vi "MH_WriteTestPTUFile.vi"(8 "entrée d'erreur":errorcluster) -> (0 "sortie d'erreur":errorcluster, 3 "refnum Out":refnum<file>)   [LabVIEW 2019]
panel:
  out "Tableau":u32[](array[numeric])
  in  "Path":path
  in  "TagArray":T1(array[cluster])=[{"TagIdent"="File_GUID", "TagIndex"=-1, "TagType"=1073872895, "TagValue"=40, "TagAuxData"="{197B8EE0-02FE-45EA-A6B5-3F8BBDE2D882}\u0000\u0000"}, {"TagIdent"="File_AssuredContent", "TagIndex"=-1, "TagType"=1073872895, "TagValue"=32, "TagAuxData"="MultiHarp: HWSETG SWSETG\u0000\u0000\u0000\u0000\u0000\u0000\u0000\u0000"}, {"TagIdent"="CreatorSW_ContentVersion", "TagIndex"=-1, "TagType"=1073872895, "TagValue"=8, "TagAuxData"="1.0\u0000\u0000\u0000\u0000\u0000"}, {"TagIdent"="CreatorSW_Name", "TagIndex"=-1, "TagType"=1073872895, "TagValue"=16, "TagAuxData"="MultiHarp AcqUI\u0000"}, {"TagIdent"="CreatorSW_Version", "TagIndex"=-1, "TagType"=1073872895, "TagValue"=8, "TagAuxData"="3.0.0.0\u0000"}, {"TagIdent"="File_CreatingTime", "TagIndex"=-1, "TagType"=553648136, "TagValue"=4676398420989345414, "TagAuxData"=""}, {"TagIdent"="File_Comment", "TagIndex"=-1, "TagType"=1073872895, "TagValue"=8, "TagAuxData"="T2 Mode\u0000"}, {"TagIdent"="Measurement_Mode", "TagIndex"=-1, "TagType"=268435464, "TagValue"=2, "TagAuxData"=""}, {"TagIdent"="Measurement_SubMode", "TagIndex"=-1, "TagType"=268435464, "TagValue"=0, "TagAuxData"=""}, {"TagIdent"="TTResult_StopReason", "TagIndex"=-1, "TagType"=268435464, "TagValue"=0, "TagAuxData"=""}, {"TagIdent"="Fast_Load_End", "TagIndex"=-1, "TagType"=-65528, "TagValue"=0, "TagAuxData"=""}, {"TagIdent"="TTResultFormat_TTTRRecType", "TagIndex"=-1, "TagType"=268435464, "TagValue"=66055, "TagAuxData"=""}, {"TagIdent"="TTResultFormat_BitsPerRecord", "TagIndex"=-1, "TagType"=268435464, "TagValue"=32, "TagAuxData"=""}, {"TagIdent"="MeasDesc_BinningFactor", "TagIndex"=-1, "TagType"=268435464, "TagValue"=32, "TagAuxData"=""}, {"TagIdent"="MeasDesc_Offset", "TagIndex"=-1, "TagType"=268435464, "TagValue"=0, "TagAuxData"=""}, {"TagIdent"="MeasDesc_AcquisitionTime", "TagIndex"=-1, "TagType"=268435464, "TagValue"=900000, "TagAuxData"=""}, {"TagIdent"="MeasDesc_StopAt", "TagIndex"=-1, "TagType"=268435464, "TagValue"=4294967295, "TagAuxData"=""}, {"TagIdent"="MeasDesc_StopOnOvfl", "TagIndex"=-1, "TagType"=8, "TagValue"=0, "TagAuxData"=""}, {"TagIdent"="MeasDesc_Restart", "TagIndex"=-1, "TagType"=8, "TagValue"=0, "TagAuxData"=""}, {"TagIdent"="CurSWSetting_DispLog", "TagIndex"=-1, "TagType"=8, "TagValue"=-1, "TagAuxData"=""}, {"TagIdent"="CurSWSetting_DispAxisTimeFrom", "TagIndex"=-1, "TagType"=268435464, "TagValue"=1, "TagAuxData"=""}, {"TagIdent"="CurSWSetting_DispAxisTimeTo", "TagIndex"=-1, "TagType"=268435464, "TagValue"=120, "TagAuxData"=""}, {"TagIdent"="CurSWSetting_DispAxisCountFrom", "TagIndex"=-1, "TagType"=268435464, "TagValue"=1, "TagAuxData"=""}, {"TagIdent"="CurSWSetting_DispAxisCountTo", "TagIndex"=-1, "TagType"=268435464, "TagValue"=10000, "TagAuxData"=""}, {"TagIdent"="CurSWSetting_DispCurves", "TagIndex"=-1, "TagType"=268435464, "TagValue"=16, "TagAuxData"=""}, {"TagIdent"="CurSWSetting_DispCurve_MapTo", "TagIndex"=0, "TagType"=268435464, "TagValue"=0, "TagAuxData"=""}, {"TagIdent"="CurSWSetting_DispCurve_Show", "TagIndex"=0, "TagType"=8, "TagValue"=-1, "TagAuxData"=""}, {"TagIdent"="CurSWSetting_DispCurve_MapTo", "TagIndex"=1, "TagType"=268435464, "TagValue"=1, "TagAuxData"=""}, {"TagIdent"="CurSWSetting_DispCurve_Show", "TagIndex"=1, "TagType"=8, "TagValue"=-1, "TagAuxData"=""}, {"TagIdent"="CurSWSetting_DispCurve_MapTo", "TagIndex"=2, "TagType"=268435464, "TagValue"=2, "TagAuxData"=""}, {"TagIdent"="CurSWSetting_DispCurve_Show", "TagIndex"=2, "TagType"=8, "TagValue"=-1, "TagAuxData"=""}, {"TagIdent"="CurSWSetting_DispCurve_MapTo", "TagIndex"=3, "TagType"=268435464, "TagValue"=3, "TagAuxData"=""}, {"TagIdent"="CurSWSetting_DispCurve_Show", "TagIndex"=3, "TagType"=8, "TagValue"=-1, "TagAuxData"=""}, {"TagIdent"="CurSWSetting_DispCurve_MapTo", "TagIndex"=4, "TagType"=268435464, "TagValue"=4, "TagAuxData"=""}, {"TagIdent"="CurSWSetting_DispCurve_Show", "TagIndex"=4, "TagType"=8, "TagValue"=-1, "TagAuxData"=""}, {"TagIdent"="CurSWSetting_DispCurve_MapTo", "TagIndex"=5, "TagType"=268435464, "TagValue"=5, "TagAuxData"=""}, {"TagIdent"="CurSWSetting_DispCurve_Show", "TagIndex"=5, "TagType"=8, "TagValue"=-1, "TagAuxData"=""}, {"TagIdent"="CurSWSetting_DispCurve_MapTo", "TagIndex"=6, "TagType"=268435464, "TagValue"=6, "TagAuxData"=""}, {"TagIdent"="CurSWSetting_DispCurve_Show", "TagIndex"=6, "TagType"=8, "TagValue"=-1, "TagAuxData"=""}, {"TagIdent"="CurSWSetting_DispCurve_MapTo", "TagIndex"=7, "TagType"=268435464, "TagValue"=7, "TagAuxData"=""}, {"TagIdent"="CurSWSetting_DispCurve_Show", "TagIndex"=7, "TagType"=8, "TagValue"=-1, "TagAuxData"=""}, {"TagIdent"="CurSWSetting_DispCurve_MapTo", "TagIndex"=8, "TagType"=268435464, "TagValue"=8, "TagAuxData"=""}, {"TagIdent"="CurSWSetting_DispCurve_Show", "TagIndex"=8, "TagType"=8, "TagValue"=-1, "TagAuxData"=""}, {"TagIdent"="CurSWSetting_DispCurve_MapTo", "TagIndex"=9, "TagType"=268435464, "TagValue"=9, "TagAuxData"=""}, {"TagIdent"="CurSWSetting_DispCurve_Show", "TagIndex"=9, "TagType"=8, "TagValue"=-1, "TagAuxData"=""}, {"TagIdent"="CurSWSetting_DispCurve_MapTo", "TagIndex"=10, "TagType"=268435464, "TagValue"=10, "TagAuxData"=""}, {"TagIdent"="CurSWSetting_DispCurve_Show", "TagIndex"=10, "TagType"=8, "TagValue"=-1, "TagAuxData"=""}, {"TagIdent"="CurSWSetting_DispCurve_MapTo", "TagIndex"=11, "TagType"=268435464, "TagValue"=11, "TagAuxData"=""}, {"TagIdent"="CurSWSetting_DispCurve_Show", "TagIndex"=11, "TagType"=8, "TagValue"=-1, "TagAuxData"=""}, {"TagIdent"="CurSWSetting_DispCurve_MapTo", "TagIndex"=12, "TagType"=268435464, "TagValue"=12, "TagAuxData"=""}, {"TagIdent"="CurSWSetting_DispCurve_Show", "TagIndex"=12, "TagType"=8, "TagValue"=-1, "TagAuxData"=""}, {"TagIdent"="CurSWSetting_DispCurve_MapTo", "TagIndex"=13, "TagType"=268435464, "TagValue"=13, "TagAuxData"=""}, {"TagIdent"="CurSWSetting_DispCurve_Show", "TagIndex"=13, "TagType"=8, "TagValue"=-1, "TagAuxData"=""}, {"TagIdent"="CurSWSetting_DispCurve_MapTo", "TagIndex"=14, "TagType"=268435464, "TagValue"=14, "TagAuxData"=""}, {"TagIdent"="CurSWSetting_DispCurve_Show", "TagIndex"=14, "TagType"=8, "TagValue"=-1, "TagAuxData"=""}, {"TagIdent"="CurSWSetting_DispCurve_MapTo", "TagIndex"=15, "TagType"=268435464, "TagValue"=15, "TagAuxData"=""}, {"TagIdent"="CurSWSetting_DispCurve_Show", "TagIndex"=15, "TagType"=8, "TagValue"=-1, "TagAuxData"=""}, {"TagIdent"="HW_Type", "TagIndex"=-1, "TagType"=1073872895, "TagValue"=24, "TagAuxData"="MultiHarp 150 4P\u0000\u0000\u0000\u0000\u0000\u0000\u0000\u0000"}, {"TagIdent"="HW_PartNo", "TagIndex"=-1, "TagType"=1073872895, "TagValue"=8, "TagAuxData"="930043\u0000\u0000"}, {"TagIdent"="HW_Version", "TagIndex"=-1, "TagType"=1073872895, "TagValue"=8, "TagAuxData"="1.0\u0000\u0000\u0000\u0000\u0000"}, {"TagIdent"="HW_SerialNo", "TagIndex"=-1, "TagType"=1073872895, "TagValue"=8, "TagAuxData"="1043897\u0000"}, {"TagIdent"="HW_Features", "TagIndex"=-1, "TagType"=285212680, "TagValue"=183, "TagAuxData"=""}, {"TagIdent"="HW_BaseResolution", "TagIndex"=-1, "TagType"=536870920, "TagValue"=4437731733528994965, "TagAuxData"=""}, {"TagIdent"="HW_InpChannels", "TagIndex"=-1, "TagType"=268435464, "TagValue"=4, "TagAuxData"=""}, {"TagIdent"="HW_ExternalRefClock", "TagIndex"=-1, "TagType"=8, "TagValue"=0, "TagAuxData"=""}, {"TagIdent"="HW_ExternalDevices", "TagIndex"=-1, "TagType"=268435464, "TagValue"=0, "TagAuxData"=""}, {"TagIdent"="HWTriggerOut_Period", "TagIndex"=-1, "TagType"=536870920, "TagValue"=4502148214488346441, "TagAuxData"=""}, {"TagIdent"="HWTriggerOut_On", "TagIndex"=-1, "TagType"=8, "TagValue"=0, "TagAuxData"=""}, {"TagIdent"="HW_InputHysteresis", "TagIndex"=-1, "TagType"=8, "TagValue"=0, "TagAuxData"=""}, {"TagIdent"="HWSync_Divider", "TagIndex"=-1, "TagType"=268435464, "TagValue"=1, "TagAuxData"=""}, {"TagIdent"="HWSync_TrgLevel", "TagIndex"=-1, "TagType"=268435464, "TagValue"=-10, "TagAuxData"=""}, {"TagIdent"="HWSync_TrgEdge", "TagIndex"=-1, "TagType"=268435464, "TagValue"=0, "TagAuxData"=""}, {"TagIdent"="HWSync_Offset", "TagIndex"=-1, "TagType"=268435464, "TagValue"=27000, "TagAuxData"=""}, {"TagIdent"="HWSync_TdCode", "TagIndex"=-1, "TagType"=268435464, "TagValue"=0, "TagAuxData"=""}, {"TagIdent"="HWInpChan_TrgLevel", "TagIndex"=0, "TagType"=268435464, "TagValue"=-150, "TagAuxData"=""}, {"TagIdent"="HWInpChan_TrgEdge", "TagIndex"=0, "TagType"=268435464, "TagValue"=0, "TagAuxData"=""}, {"TagIdent"="HWInpChan_Offset", "TagIndex"=0, "TagType"=268435464, "TagValue"=0, "TagAuxData"=""}, {"TagIdent"="HWInpChan_Enabled", "TagIndex"=0, "TagType"=8, "TagValue"=-1, "TagAuxData"=""}, {"TagIdent"="HWInpChan_TdCode", "TagIndex"=0, "TagType"=268435464, "TagValue"=0, "TagAuxData"=""}, {"TagIdent"="HWInpChan_TrgLevel", "TagIndex"=1, "TagType"=268435464, "TagValue"=-150, "TagAuxData"=""}, {"TagIdent"="HWInpChan_TrgEdge", "TagIndex"=1, "TagType"=268435464, "TagValue"=0, "TagAuxData"=""}, {"TagIdent"="HWInpChan_Offset", "TagIndex"=1, "TagType"=268435464, "TagValue"=0, "TagAuxData"=""}, {"TagIdent"="HWInpChan_Enabled", "TagIndex"=1, "TagType"=8, "TagValue"=-1, "TagAuxData"=""}, {"TagIdent"="HWInpChan_TdCode", "TagIndex"=1, "TagType"=268435464, "TagValue"=0, "TagAuxData"=""}, {"TagIdent"="HWInpChan_TrgLevel", "TagIndex"=2, "TagType"=268435464, "TagValue"=-50, "TagAuxData"=""}, {"TagIdent"="HWInpChan_TrgEdge", "TagIndex"=2, "TagType"=268435464, "TagValue"=0, "TagAuxData"=""}, {"TagIdent"="HWInpChan_Offset", "TagIndex"=2, "TagType"=268435464, "TagValue"=0, "TagAuxData"=""}, {"TagIdent"="HWInpChan_Enabled", "TagIndex"=2, "TagType"=8, "TagValue"=-1, "TagAuxData"=""}, {"TagIdent"="HWInpChan_TdCode", "TagIndex"=2, "TagType"=268435464, "TagValue"=0, "TagAuxData"=""}, {"TagIdent"="HWInpChan_TrgLevel", "TagIndex"=3, "TagType"=268435464, "TagValue"=-50, "TagAuxData"=""}, {"TagIdent"="HWInpChan_TrgEdge", "TagIndex"=3, "TagType"=268435464, "TagValue"=0, "TagAuxData"=""}, {"TagIdent"="HWInpChan_Offset", "TagIndex"=3, "TagType"=268435464, "TagValue"=0, "TagAuxData"=""}, {"TagIdent"="HWInpChan_Enabled", "TagIndex"=3, "TagType"=8, "TagValue"=-1, "TagAuxData"=""}, {"TagIdent"="HWInpChan_TdCode", "TagIndex"=3, "TagType"=268435464, "TagValue"=0, "TagAuxData"=""}, {"TagIdent"="MeasDesc_Resolution", "TagIndex"=-1, "TagType"=536870920, "TagValue"=4437731733528994965, "TagAuxData"=""}, {"TagIdent"="HW_Markers", "TagIndex"=-1, "TagType"=268435464, "TagValue"=4, "TagAuxData"=""}, {"TagIdent"="HWMarkers_RisingEdge", "TagIndex"=0, "TagType"=8, "TagValue"=0, "TagAuxData"=""}, {"TagIdent"="HWMarkers_RisingEdge", "TagIndex"=1, "TagType"=8, "TagValue"=0, "TagAuxData"=""}, {"TagIdent"="HWMarkers_RisingEdge", "TagIndex"=2, "TagType"=8, "TagValue"=0, "TagAuxData"=""}, {"TagIdent"="HWMarkers_RisingEdge", "TagIndex"=3, "TagType"=8, "TagValue"=0, "TagAuxData"=""}, {"TagIdent"="HWMarkers_Enabled", "TagIndex"=0, "TagType"=8, "TagValue"=-1, "TagAuxData"=""}, {"TagIdent"="HWMarkers_Enabled", "TagIndex"=1, "TagType"=8, "TagValue"=-1, "TagAuxData"=""}, {"TagIdent"="HWMarkers_Enabled", "TagIndex"=2, "TagType"=8, "TagValue"=-1, "TagAuxData"=""}, {"TagIdent"="HWMarkers_Enabled", "TagIndex"=3, "TagType"=8, "TagValue"=-1, "TagAuxData"=""}, {"TagIdent"="HWMarkers_HoldOff", "TagIndex"=-1, "TagType"=268435464, "TagValue"=0, "TagAuxData"=""}, {"TagIdent"="MeasDesc_GlobalResolution", "TagIndex"=-1, "TagType"=536870920, "TagValue"=4437731733528994965, "TagAuxData"=""}, {"TagIdent"="TTResult_SyncRate", "TagIndex"=-1, "TagType"=268435464, "TagValue"=0, "TagAuxData"=""}, {"TagIdent"="TTResult_InputRate", "TagIndex"=0, "TagType"=268435464, "TagValue"=9126, "TagAuxData"=""}, {"TagIdent"="TTResult_InputRate", "TagIndex"=1, "TagType"=268435464, "TagValue"=8247, "TagAuxData"=""}, {"TagIdent"="TTResult_InputRate", "TagIndex"=2, "TagType"=268435464, "TagValue"=0, "TagAuxData"=""}, {"TagIdent"="TTResult_InputRate", "TagIndex"=3, "TagType"=268435464, "TagValue"=0, "TagAuxData"=""}, {"TagIdent"="TTResult_StopAfter", "TagIndex"=-1, "TagType"=268435464, "TagValue"=900000, "TagAuxData"=""}, {"TagIdent"="TTResult_NumberOfRecords", "TagIndex"=-1, "TagType"=268435464, "TagValue"=10000, "TagAuxData"=""}, {"TagIdent"="TTResult_MDescWarningFlags", "TagIndex"=-1, "TagType"=285212680, "TagValue"=0, "TagAuxData"=""}, {"TagIdent"="Header_End", "TagIndex"=-1, "TagType"=-65528, "TagValue"=0, "TagAuxData"=""}]
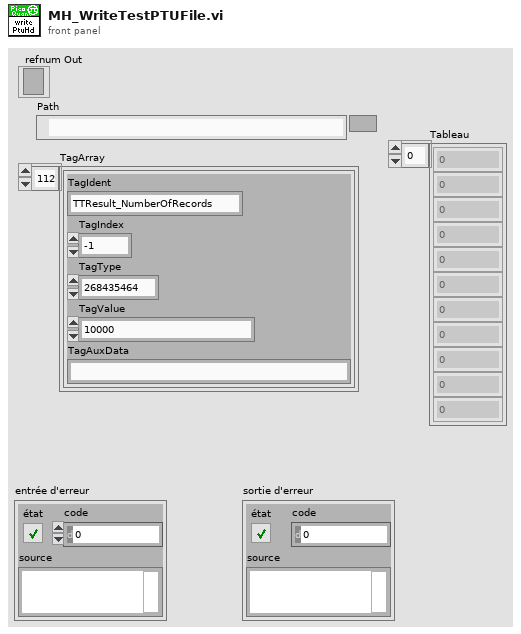
[diagram p1: front panel]
types:
  T1 = cluster{"TagIdent":string, "TagIndex":i32, "TagType":i32, "TagValue":i64, "TagAuxData":string}[]
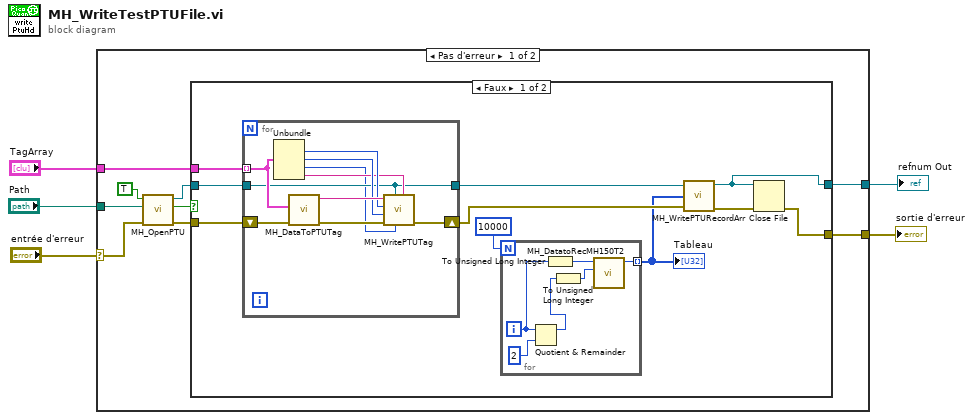
[diagram p0: block diagram]
diagram:
  n1 = case shown="Pas d'erreur" "entrée d'erreur" {
    selector: "entrée d'erreur" -> [w11 w43]
    tunnel: [w14 w43] -> w5
    tunnel: "Path" -> [w9 _]
    tunnel: "TagArray" -> [w7 _]
    tunnel: [w6 _] -> w1
    frame No Error {
      n2 = call <userlib>:"MH_OpenPTU.vi"("ErrorIn"=w11, "chemin sélectionné"=w9, "WriteMode"=TRUE) -> ("ErrorOut"=w12:errorcluster, "Cancelled"=w8:bool, "refnum en sortie"=w13:refnum<file>)  [unwired: 6 in]
      n3 = case shown="Faux" w8 {
        tunnel: w12 -> [w23 w42]
        tunnel: [w21 w42] -> w14
        tunnel: w13 -> [w22 w41]
        tunnel: w7 -> [w24 _]
        tunnel: [w15 w41] -> w6
        frame False {
          n4 = for {
            tunnel: w24 -> [w40] mode=indexing
            shift-right: [w33] -> w18
            shift-left: w23 -> [w34]
            tunnel: w22 -> [w32]
            tunnel: [w32] -> w17
            n5 = Unbundle(w40) -> ("TagIndex"=w38:i32, "TagType"=w37:i32, "TagValue"=w31:i64, "TagAuxData"=w36:string)  [unwired: 1 out]
            n6 = call <userlib>:"MH_DataToPTUTag.vi"("error in"=w34, "TagIn"=w40) -> ("error in 2"=w35:errorcluster, "TagIdent Out"=w39:string)  [unwired: 5 in, 3 out]
            n7 = call <userlib>:"MH_WritePTUTag.vi"("TagAuxData"=w36, "TagValue"=w31, "refnum"=w32, "error in"=w35, "TagType"=w37, "TagIndex"=w38, "identifierfull"=w39) -> ("error out"=w33:errorcluster)  [unwired: 3 in]
          }
          n8 = for {
            N: 10000 -> [_]
            tunnel: [w25] -> w16 mode=indexing
            i -> [w26]
            n9 = Quotient & Remainder(x=w26, y=2) -> (x-y*floor(x/y)=w27:i32)  [unwired: 1 out]
            n10 = To Unsigned Long Integer(number=w26) -> (unsigned 32bit integer=w29:u32)
            n11 = To Unsigned Long Integer(number=w27) -> (unsigned 32bit integer=w30:u32)
            n12 = call <userlib>:"MH_DatatoRecMH150T2.vi"("channel"=w30, "Time"=w29) -> ("rawbits"=w25:u32)  [unwired: 9 in]
          }
          "Tableau" <- w16
          n13 = call <userlib>:"MH_WritePTURecordArr.vi"("refnum"=w17, "TTTR Records"=w16, "error in"=w18) -> ("refnum en sortie"=w15:refnum<file>, "error out"=w19:errorcluster)  [unwired: 6 in]
          n14 = Close File(refnum=w15, error in=w19) -> (error out=w21:errorcluster)  [unwired: 1 out]
        }
        frame True {
        }
      }
    }
    frame Error {
    }
  }
  "sortie d'erreur" <- w5
  "refnum Out" <- w1
